vi "main.vi"() -> ()   [LabVIEW 2026]
uses:
  Control/Ctrl_IndicadoresMainPanel.ctl
  Control/Ctr_Enc_Values.ctl
  Control/Ctrl_Motores_Valores.ctl
  Control/Ctrl_Errores.ctl
  Control/Ctrl_DataLoggerQueue.ctl
  Ctrl_Estados.ctl
  Control/Ctrl_EscrituraComandos.ctl
  Control/Ctrl_DLQueue.ctl
  Control/Ctrl_Fgv_DatosMotores.ctl
panel:
  out "Serial errors":u32
  in  "PWM":dbl
  in  "HomeToHome":bool
  in  "Vueltas10":bool
  in  "Serial":refnum<visa-resource-name>
  in  "Refresh Square":bool
  out "status_serial":bool
  out "Start_ind":bool
  in  "Stop Button":bool
  in  "Start Button":bool
  out "Vel_antebrazo":i32 caption="Velocidad"
  out "Vel_hombro":i32 caption="Velocidad"
  out "Vel_mun":i32 caption="Velocidad"
  out "Vel_codo":i32 caption="Velocidad"
  out "Vel_cad":i32 caption="Velocidad"
  out "V_ant":i32 caption="Vueltas"
  out "P_ant":i32 caption="Pasos"
  out "V_hombro":i32 caption="Vueltas"
  out "P_hombro":i32 caption="Pasos"
  out "V_mun":i32 caption="Vueltas"
  out "P_mun":i32 caption="Pasos"
  out "V_cod":i32 caption="Vueltas"
  out "P_cod":i32 caption="Pasos"
  out "V_cad":i32 caption="Vueltas"
  out "P_cad":i32 caption="Pasos"
  out "Enc_Muneca":i32(knob) caption="Enc. Muñeca" scale=0.0..400.0
  out "Error_out":errorcluster
  out "Corriente":dbl
  out "Voltaje":dbl
  out "Enc_Antebrazo":i32(knob) caption="Enc. Antebrazo" scale=0.0..400.0
  out "Enc_Codo":i32(knob) caption="Enc. Codo" scale=0.0..400.0
  out "Enc_Hombro":i32(knob) caption="Enc. Hombro" scale=0.0..400.0
  out "Enc_Cadera":i32(knob) caption="Enc. Cadera" scale=0.0..400.0
  # "Universidad Anáhuac Oaxaca"
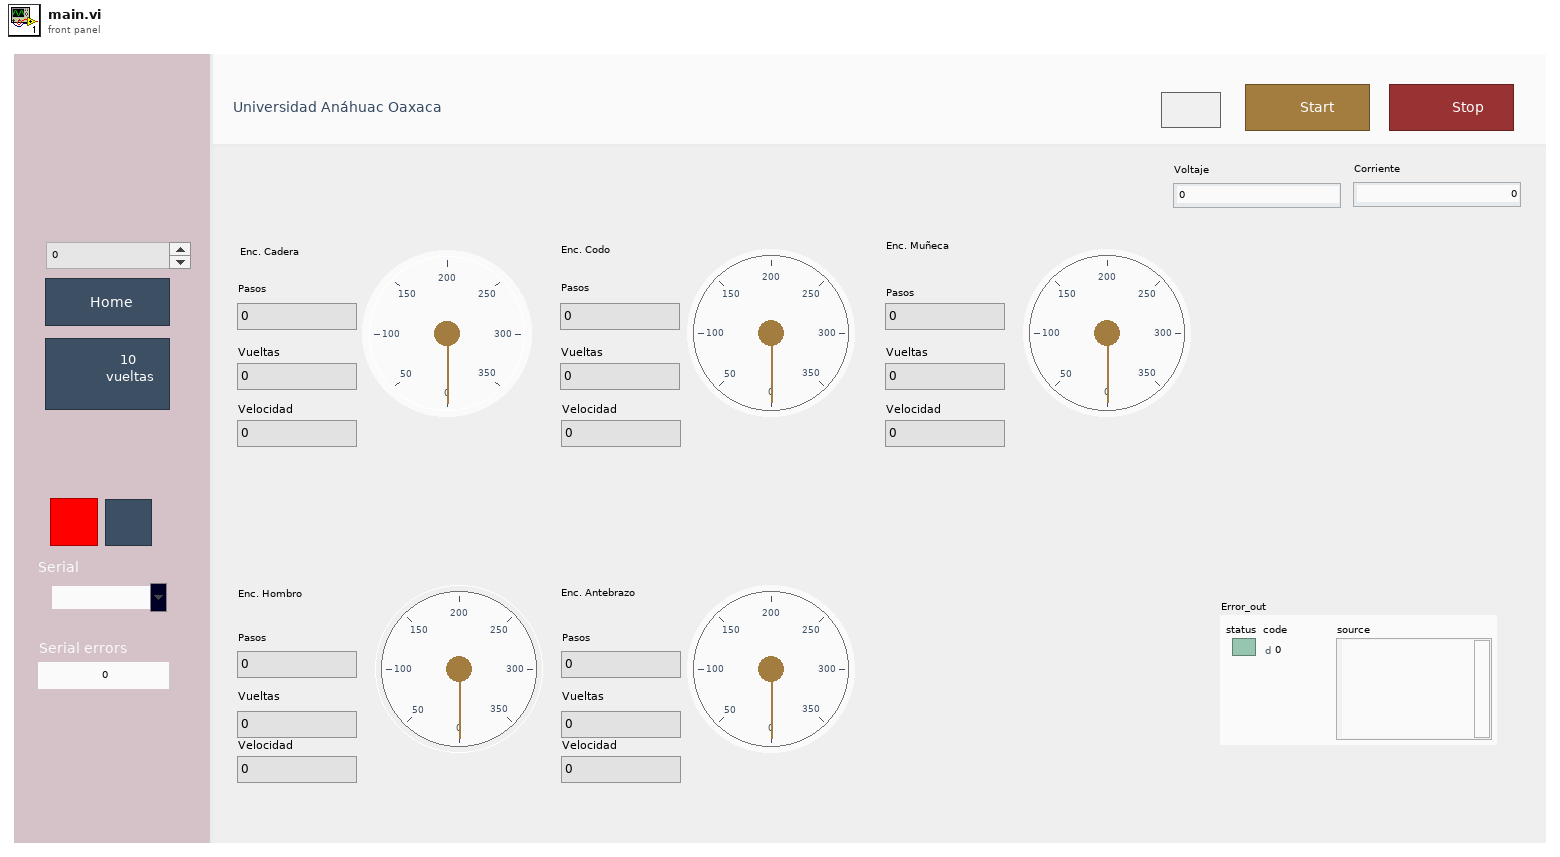
[diagram p1: front panel]
types:
  T1 = enum8{"Enabled", "Disabled", "Disabled and Grayed Out"}
  T2 = typedef "Ctr_Enc_Values.ctl" = cluster{"buffer":string, "Datos6_Motores":cluster{"M_cadera":T3, "M_hombro":T3, "M_codo":T3, "M_antebrazo":T3, "M_muneca":T3, "M_gripper":T3}, "Errores":T4, "new_data?":bool}
  T3 = typedef "Ctrl_Motores_Valores.ctl" = cluster{"Pasos":i32, "Vueltas":i16, "Velocidad":i16, "Reserva1":u8, "Reserva2":u8}
  T4 = typedef "Ctrl_Errores.ctl" = cluster{"Contador_correcto":u32, "Contador_errores":u32, "Edo_conex":u32}
  T5 = typedef "Ctrl_Fgv_DatosMotores.ctl" = enum16{"Stop", "Get", "Set"}
  T6 = typedef "Ctrl_Estados.ctl" = enum16{"LogData", "Idle", "Stop", "IDLE", "Reconnect", "Log_Data_All", "Start", "WRITE_DATA", "SEND_COM"}
  T7 = typedef "Ctrl_DLQueue.ctl" = cluster{"Estado":T6, "IncioPrograma":bool}
  T8 = typedef "Ctrl_DataLoggerQueue.ctl" = cluster{"IncioPrograma":bool, "Estado":T6, "Enc_values":T2, "Com_Escribir":T9}
  T9 = typedef "Ctrl_EscrituraComandos.ctl" = enum16{"MOVE_10", "HOME_TO"}
  T10 = typedef "Ctrl_IndicadoresMainPanel.ctl" = cluster{"status_serial":refnum<vi>, "Vel_cad":refnum<vi>, "Vel_antebrazo":refnum<vi>, "Vel_hombro":refnum<vi>, "Vel_mun":refnum<vi>, "Vel_codo":refnum<vi>, "P_mun":refnum<vi>, "P_ant":refnum<vi>, "P_cod":refnum<vi>, "P_hombro":refnum<vi>, "P_cad":refnum<vi>, "Enc_Antebrazo":refnum<vi>, "Enc_Codo":refnum<vi>, "Enc_Muneca":refnum<vi>, "Enc_Hombro":refnum<vi>, "Enc_Cadera":refnum<vi>, "V_mun":refnum<vi>, "V_ant":refnum<vi>, "V_hombro":refnum<vi>, "V_cod":refnum<vi>, "V_cad":refnum<vi>}
  T11 = enum16{"open", "replace", "create", "open or create", "replace or create", "replace or create with confirmation"}
  T12 = cluster{"M_cadera":T3, "M_hombro":T3, "M_codo":T3, "M_antebrazo":T3, "M_muneca":T3, "M_gripper":T3}
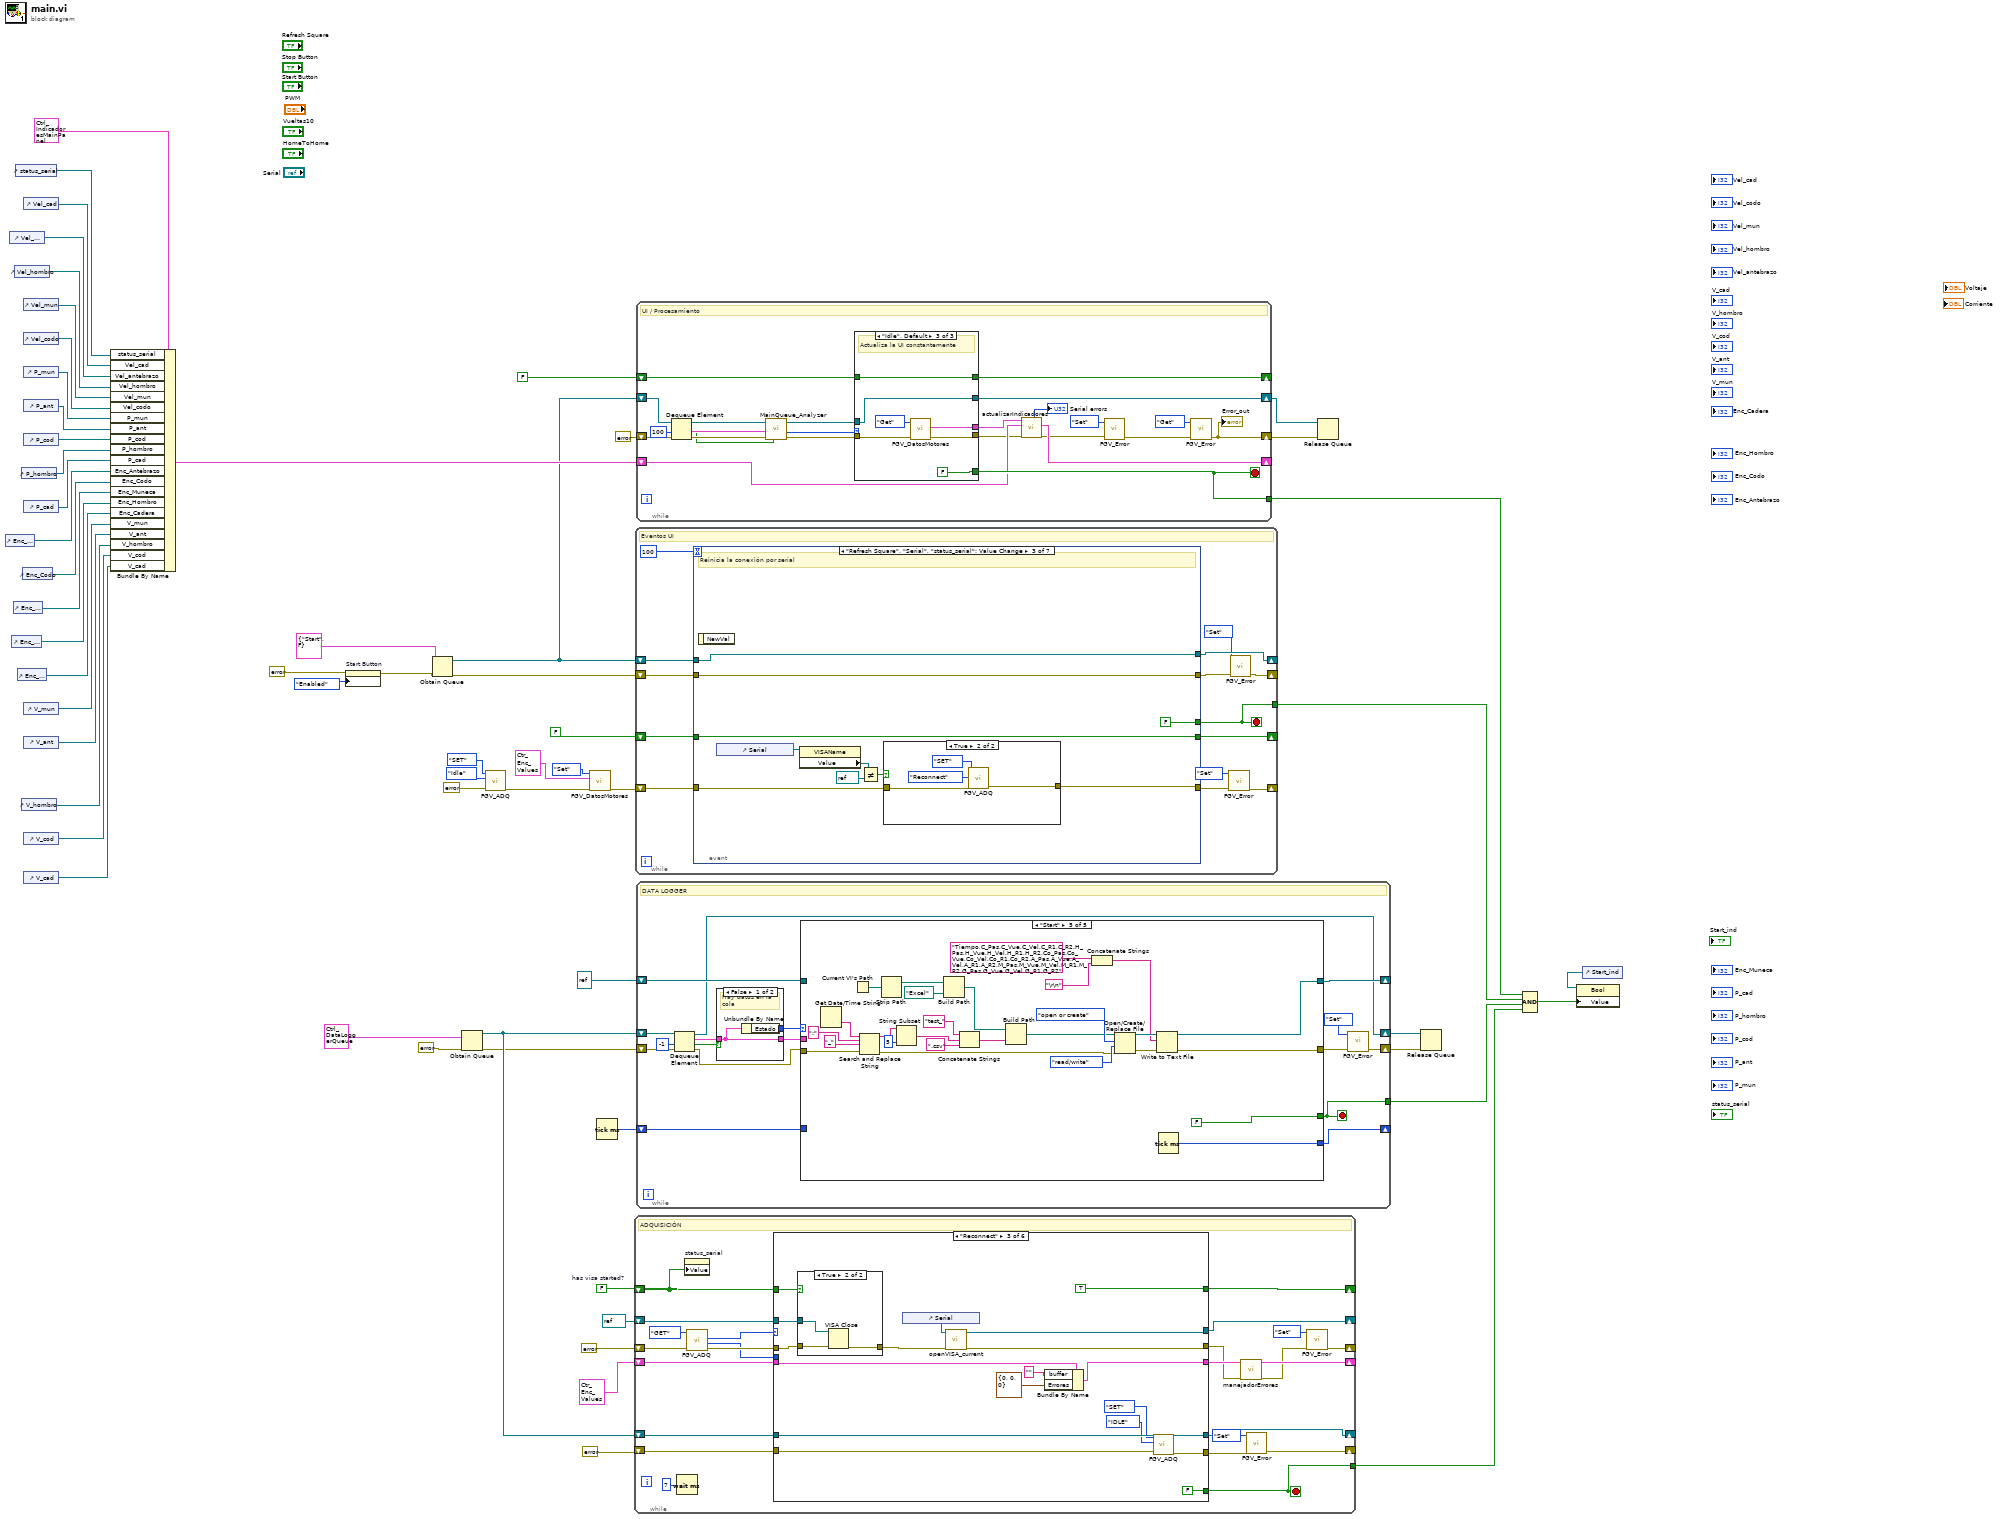
[diagram p0: block diagram]
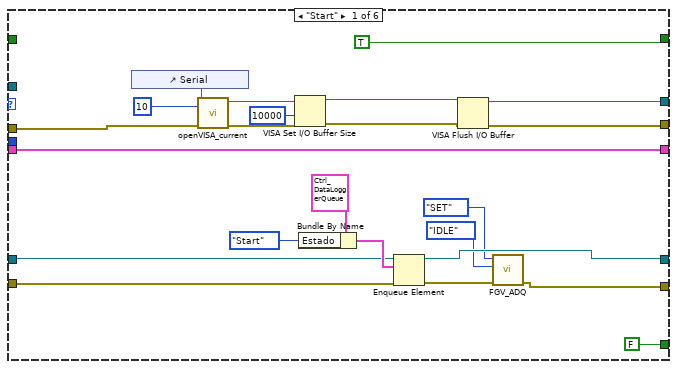
[diagram p2: hidden frame]
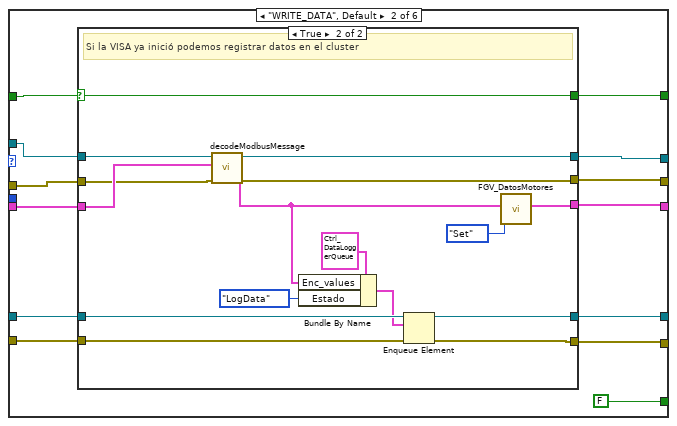
[diagram p3: hidden frame]
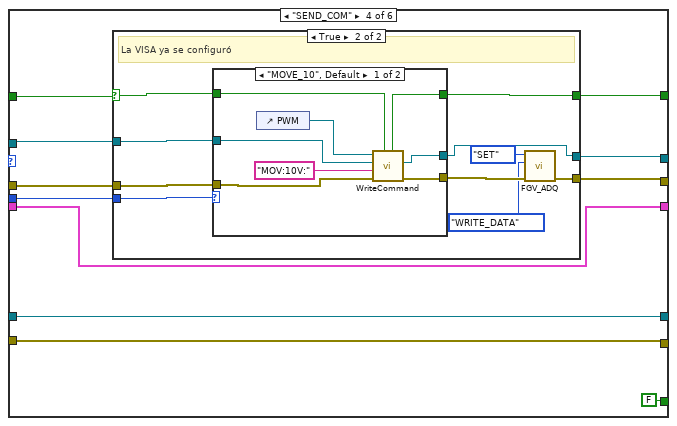
[diagram p6: hidden frame]
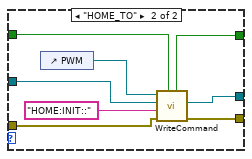
[diagram p8: hidden frame]
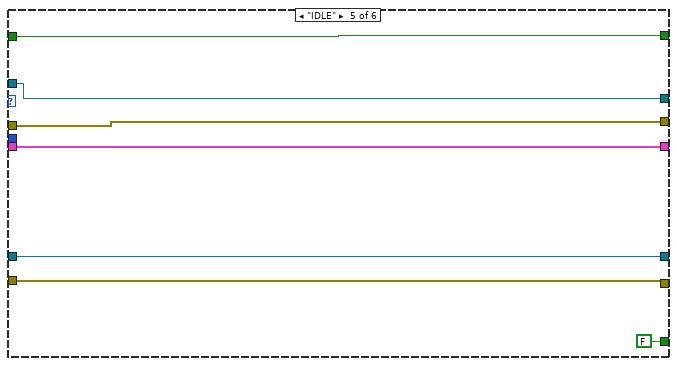
[diagram p9: hidden frame]
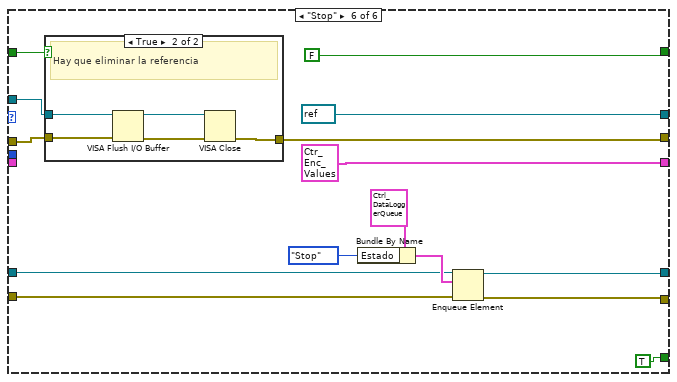
[diagram p10: hidden frame]
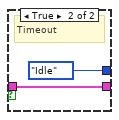
[diagram p12: hidden frame]
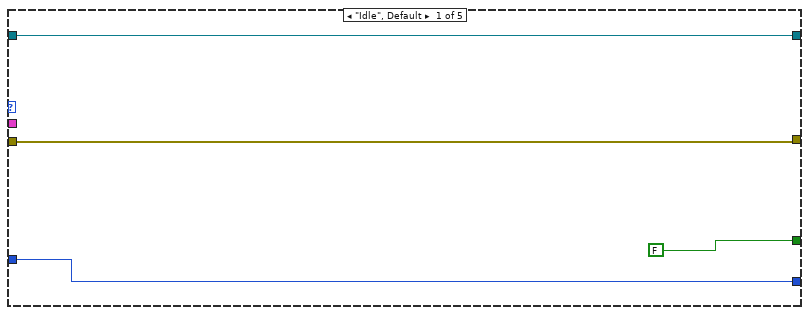
[diagram p13: hidden frame]
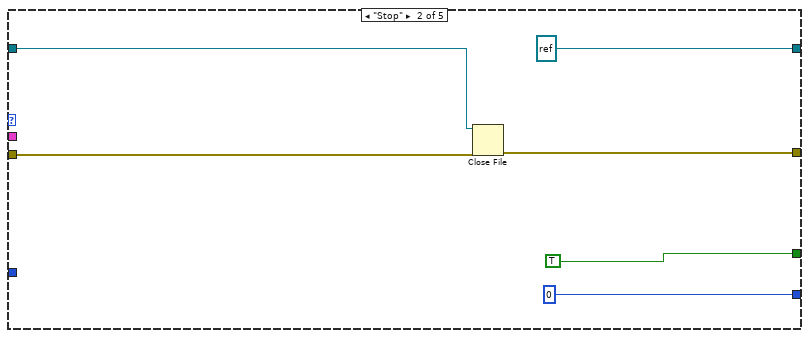
[diagram p14: hidden frame]
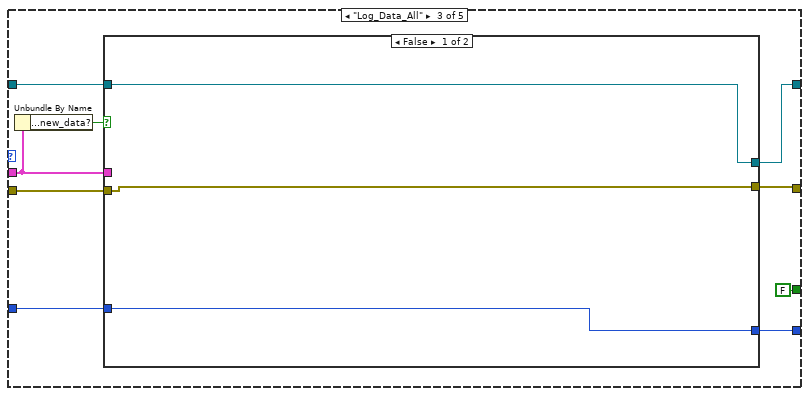
[diagram p15: hidden frame]
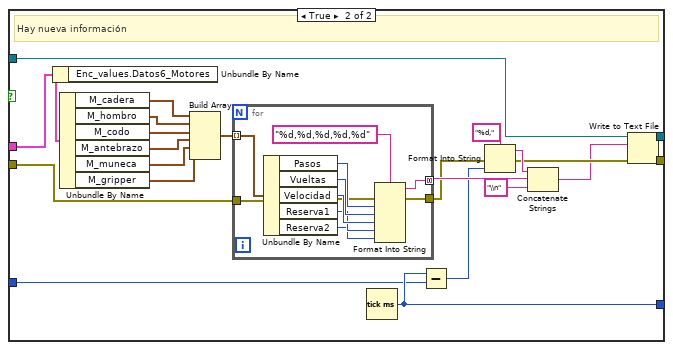
[diagram p16: hidden frame]
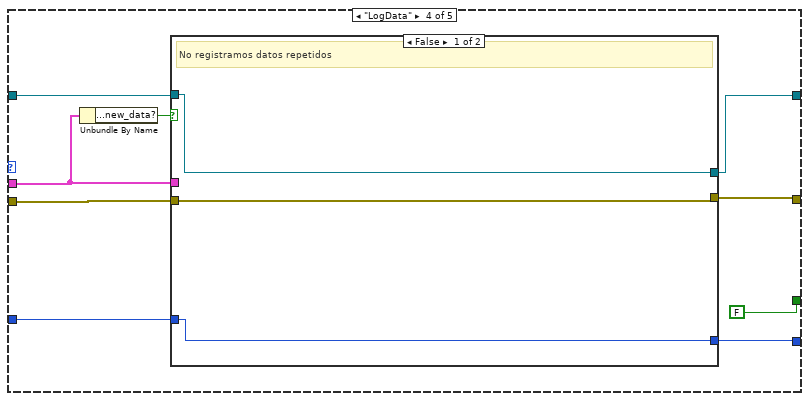
[diagram p17: hidden frame]
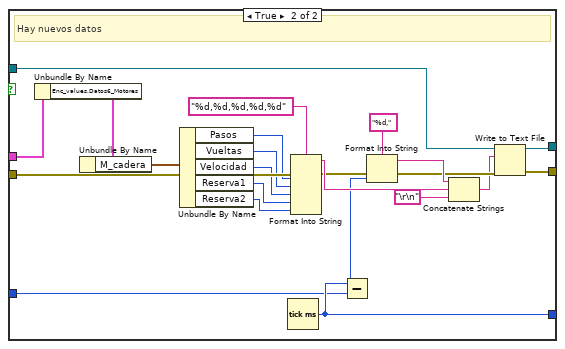
[diagram p18: hidden frame]
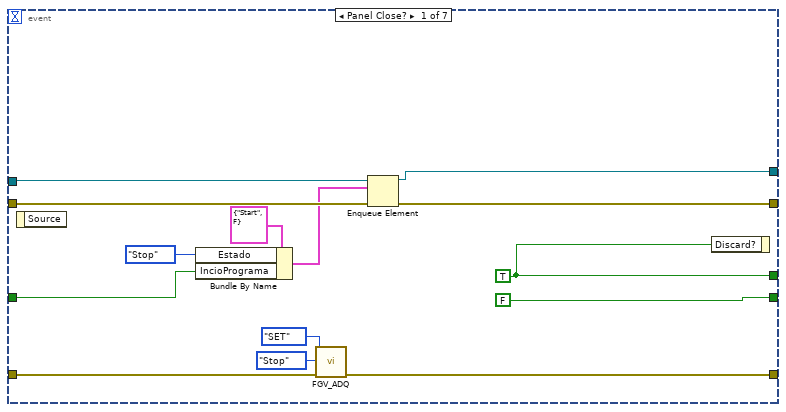
[diagram p19: hidden frame]
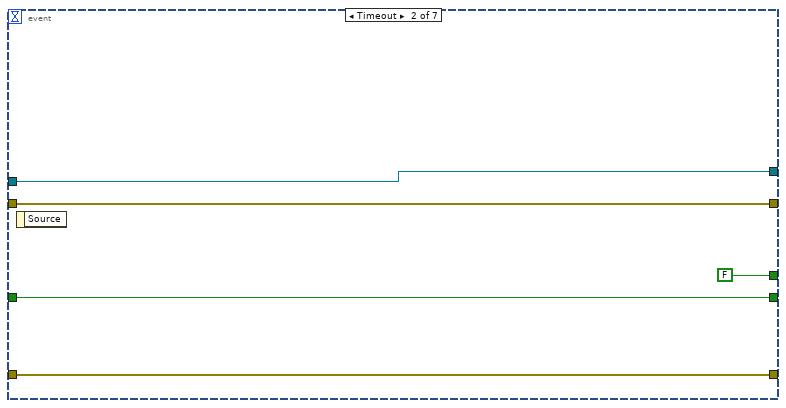
[diagram p20: hidden frame]
diagram:
  w32 = FALSE  # has visa started?
  n1 = control-ref of="Enc_Antebrazo"() -> (w47:refnum<vi>)
  n2 = control-ref of="Vel_antebrazo"() -> (w56:refnum<vi>)
  n3 = control-ref of="Enc_Hombro"() -> (w44:refnum<vi>)
  n4 = control-ref of="Enc_Muneca"() -> (w45:refnum<vi>)
  n5 = control-ref of="Vel_hombro"() -> (w55:refnum<vi>)
  n6 = control-ref of="status_serial"() -> (w59:refnum<vi>)
  n7 = control-ref of="Enc_Cadera"() -> (w43:refnum<vi>)
  n8 = control-ref of="P_hombro"() -> (w49:refnum<vi>)
  n9 = control-ref of="V_hombro"() -> (w40:refnum<vi>)
  n10 = control-ref of="Enc_Codo"() -> (w46:refnum<vi>)
  n11 = control-ref of="Vel_cad"() -> (w57:refnum<vi>)
  n12 = control-ref of="Vel_mun"() -> (w54:refnum<vi>)
  n13 = control-ref of="Vel_codo"() -> (w53:refnum<vi>)
  n14 = control-ref of="P_mun"() -> (w52:refnum<vi>)
  n15 = control-ref of="P_ant"() -> (w51:refnum<vi>)
  n16 = control-ref of="P_cod"() -> (w50:refnum<vi>)
  n17 = control-ref of="P_cad"() -> (w48:refnum<vi>)
  n18 = control-ref of="V_mun"() -> (w42:refnum<vi>)
  n19 = control-ref of="V_ant"() -> (w41:refnum<vi>)
  n20 = control-ref of="V_cod"() -> (w39:refnum<vi>)
  n21 = control-ref of="V_cad"() -> (w38:refnum<vi>)
  n22 = Bundle By Name(cluster=T10 {"status_serial"=refnum, "Vel_cad"=refnum, "Vel_antebrazo"=refnum, "Vel_hombro"=refnum, "Vel_mun"=refnum, "Vel_codo"=refnum, "P_mun"=refnum, "P_ant"=refnum, "P_cod"=refnum, "P_hombro"=refnum, "P_cad"=refnum, "Enc_Antebrazo"=refnum, "Enc_Codo"=refnum, "Enc_Muneca"=refnum, "Enc_Hombro"=refnum, "Enc_Cadera"=refnum, "V_mun"=refnum, "V_ant"=refnum, "V_hombro"=refnum, "V_cod"=refnum, "V_cad"=refnum} ("output cluster"), "status_serial"=w59, "Vel_cad"=w57, "Vel_antebrazo"=w56, "Vel_hombro"=w55, "Vel_mun"=w54, "Vel_codo"=w53, "P_mun"=w52, "P_ant"=w51, "P_cod"=w50, "P_hombro"=w49, "P_cad"=w48, "Enc_Antebrazo"=w47, "Enc_Codo"=w46, "Enc_Muneca"=w45, "Enc_Hombro"=w44, "Enc_Cadera"=w43, "V_mun"=w42, "V_ant"=w41, "V_hombro"=w40, "V_cod"=w39, "V_cad"=w38) -> (w37:T10)
  n23 = property on="Start Button" class="Bool"(error in=errorcluster {"status"=FALSE, "code"=0, "source"=""} ("error in (no error)"), "DisabledEnum"=T1."Enabled" ("Disabled")) -> (error out=w8:errorcluster)  [unwired: 1 in, 1 out]
  n24 = Obtain Queue(element data type=T7 {"Estado"=enum."Start", "IncioPrograma"=FALSE} ("estado_queue"), error in (no error)=w8) -> (queue out=w22:refnum<queue>, error out=w21:errorcluster)  [unwired: 3 in, 1 out]
  n25 = Obtain Queue(element data type=T8 {"IncioPrograma"=FALSE, "Estado"=enum."Start", "Enc_values"={"buffer"="", "Datos6_Motores"={"M_cadera"={"Pasos"=0, "Vueltas"=0, "Velocidad"=0, "Reserva1"=0, "Reserva2"=0}, "M_hombro"={"Pasos"=0, "Vueltas"=0, "Velocidad"=0, "Reserva1"=0, "Reserva2"=0}, "M_codo"={"Pasos"=0, "Vueltas"=0, "Velocidad"=0, "Reserva1"=0, "Reserva2"=0}, "M_antebrazo"={"Pasos"=0, "Vueltas"=0, "Velocidad"=0, "Reserva1"=0, "Reserva2"=0}, "M_muneca"={"Pasos"=0, "Vueltas"=0, "Velocidad"=0, "Reserva1"=0, "Reserva2"=0}, "M_gripper"={"Pasos"=0, "Vueltas"=0, "Velocidad"=0, "Reserva1"=0, "Reserva2"=0}}, "Errores"={"Contador_correcto"=0, "Contador_errores"=0, "Edo_conex"=0}, "new_data?"=FALSE}, "Com_Escribir"=enum."MOVE_10"} ("datalogger_cluster"), error in (no error)=errorcluster {"status"=FALSE, "code"=0, "source"=""}) -> (queue out=w10:refnum<queue>, error out=w9:errorcluster)  [unwired: 3 in, 1 out]
  n26 = call "FGV_ADQ.vi"("error in (no error)"=errorcluster {"status"=FALSE, "code"=0, "source"=""}, "SM_IN"=Ctrl_Estados."Idle", "SET/GET"=enum16{"SET", "GET"}."SET") -> ("error out"=w11:errorcluster)  [unwired: 6 in, 2 out]
  n27 = call "FGV_DatosMotores.vi"("error in (no error)"=w11, "Val_motor_in"=T2 {"buffer"="", "Datos6_Motores"={"M_cadera"={"Pasos"=0, "Vueltas"=0, "Velocidad"=0, "Reserva1"=0, "Reserva2"=0}, "M_hombro"={"Pasos"=0, "Vueltas"=0, "Velocidad"=0, "Reserva1"=0, "Reserva2"=0}, "M_codo"={"Pasos"=0, "Vueltas"=0, "Velocidad"=0, "Reserva1"=0, "Reserva2"=0}, "M_antebrazo"={"Pasos"=0, "Vueltas"=0, "Velocidad"=0, "Reserva1"=0, "Reserva2"=0}, "M_muneca"={"Pasos"=0, "Vueltas"=0, "Velocidad"=0, "Reserva1"=0, "Reserva2"=0}, "M_gripper"={"Pasos"=0, "Vueltas"=0, "Velocidad"=0, "Reserva1"=0, "Reserva2"=0}}, "Errores"={"Contador_correcto"=0, "Contador_errores"=0, "Edo_conex"=0}, "new_data?"=FALSE}, "Estado"=Ctrl_Fgv_DatosMotores."Set") -> ("error out"=w14:errorcluster)  [unwired: 7 in, 1 out]
  n28 = Tick Count (ms)() -> (millisecond timer value=w36:u32)
  n29 = while {
    shift-right: [w75] -> _
    shift-left: T2 {"buffer"="", "Datos6_Motores"={"M_cadera"={"Pasos"=0, "Vueltas"=0, "Velocidad"=0, "Reserva1"=0, "Reserva2"=0}, "M_hombro"={"Pasos"=0, "Vueltas"=0, "Velocidad"=0, "Reserva1"=0, "Reserva2"=0}, "M_codo"={"Pasos"=0, "Vueltas"=0, "Velocidad"=0, "Reserva1"=0, "Reserva2"=0}, "M_antebrazo"={"Pasos"=0, "Vueltas"=0, "Velocidad"=0, "Reserva1"=0, "Reserva2"=0}, "M_muneca"={"Pasos"=0, "Vueltas"=0, "Velocidad"=0, "Reserva1"=0, "Reserva2"=0}, "M_gripper"={"Pasos"=0, "Vueltas"=0, "Velocidad"=0, "Reserva1"=0, "Reserva2"=0}}, "Errores"={"Contador_correcto"=0, "Contador_errores"=0, "Edo_conex"=0}, "new_data?"=FALSE} ("Enc_values") -> [w84]
    shift-right: [w83] -> _
    shift-left: refnum<visa-resource-name> refnum ("VISA resource name out") -> [w81]
    shift-right: [w71] -> _
    shift-left: errorcluster {"status"=FALSE, "code"=0, "source"=""} ("error in (no error)") -> [w67]
    shift-right: [w82] -> _
    shift-left: w32 -> [w62]
    shift-right: [w64] -> _
    shift-left: errorcluster {"status"=FALSE, "code"=0, "source"=""} ("error in (no error)") -> [w80]
    shift-right: [w78] -> _
    shift-left: w10 -> [w79]
    tunnel: [w77] -> w24
    stop <- w77 stop-if-true
    # "ADQUISICIÓN"
    n30 = Wait (ms)(milliseconds to wait=u32 7) -> ()  [unwired: 1 out]
    n31 = property on="status_serial" class="Bool"("Value"=w62) -> ()  [unwired: 2 in, 2 out]
    n32 = call "FGV_ADQ.vi"("error in (no error)"=w67, "SET/GET"=enum16{"SET", "GET"}."GET") -> ("error out"=w68:errorcluster, "Com_Escribir_OUT"=w66:T9, "SM_OUT"=w69:T6)  [unwired: 7 in]
    n33 = case shown="\"Reconnect\"" w69 {
      tunnel: w84 -> [w106 w120 w154 w172 w208 _]
      tunnel: w81 -> [_ w119 w157 w175 w210 w225]
      tunnel: w62 -> [_ w117 w152 w170 w211 w226]
      tunnel: [w88 w110 w155 w174 w209 w221] -> w74
      tunnel: [w89 w118 w150 w171 w210 refnum<visa-resource-name> refnum ("VISA resource name out")] -> w83
      tunnel: [TRUE w113 TRUE ("start_out") w173 w211 FALSE] -> w82
      tunnel: [w106 w111 w153 w172 w208 T2 {"buffer"="", "Datos6_Motores"={"M_cadera"={"Pasos"=0, "Vueltas"=0, "Velocidad"=0, "Reserva1"=0, "Reserva2"=0}, "M_hombro"={"Pasos"=0, "Vueltas"=0, "Velocidad"=0, "Reserva1"=0, "Reserva2"=0}, "M_codo"={"Pasos"=0, "Vueltas"=0, "Velocidad"=0, "Reserva1"=0, "Reserva2"=0}, "M_antebrazo"={"Pasos"=0, "Vueltas"=0, "Velocidad"=0, "Reserva1"=0, "Reserva2"=0}, "M_muneca"={"Pasos"=0, "Vueltas"=0, "Velocidad"=0, "Reserva1"=0, "Reserva2"=0}, "M_gripper"={"Pasos"=0, "Vueltas"=0, "Velocidad"=0, "Reserva1"=0, "Reserva2"=0}}, "Errores"={"Contador_correcto"=0, "Contador_errores"=0, "Edo_conex"=0}, "new_data?"=FALSE} ("Enc_values")] -> w76
      tunnel: w80 -> [w101 w116 w143 w165 w205 w216]
      tunnel: w79 -> [w102 w115 w149 w169 w207 w217]
      tunnel: [w100 w114 w149 w169 w207 w215] -> w78
      tunnel: [FALSE FALSE FALSE FALSE FALSE TRUE] -> w77
      tunnel: w68 -> [w98 w109 w147 w167 w209 w213]
      tunnel: w66 -> [_ _ _ w166 _ _]
      tunnel: [w85 w108 w144 w165 w205 w212] -> w61
      frame "Start" {
        n34 = control-ref of="Serial"() -> (w107:refnum<vi>)
        n35 = call "openVISA_current.vi"("error in (no error)"=w98, "Timeout"=u32 10, "VisaRef"=w107) -> ("error out"=w92:errorcluster, "VISA Refnum out"=w93:refnum<visa-resource-name>)  [unwired: 7 in]
        n36 = VISA Set I/O Buffer Size(VISA resource name=w93, size (4096)=u32 10000, error in (no error)=w92) -> (VISA resource name out=w91:refnum<visa-resource-name>, error out=w90:errorcluster)  [unwired: 1 in]
        n37 = Bundle By Name(cluster=T8 {"IncioPrograma"=FALSE, "Estado"=enum."Start", "Enc_values"={"buffer"="", "Datos6_Motores"={"M_cadera"={"Pasos"=0, "Vueltas"=0, "Velocidad"=0, "Reserva1"=0, "Reserva2"=0}, "M_hombro"={"Pasos"=0, "Vueltas"=0, "Velocidad"=0, "Reserva1"=0, "Reserva2"=0}, "M_codo"={"Pasos"=0, "Vueltas"=0, "Velocidad"=0, "Reserva1"=0, "Reserva2"=0}, "M_antebrazo"={"Pasos"=0, "Vueltas"=0, "Velocidad"=0, "Reserva1"=0, "Reserva2"=0}, "M_muneca"={"Pasos"=0, "Vueltas"=0, "Velocidad"=0, "Reserva1"=0, "Reserva2"=0}, "M_gripper"={"Pasos"=0, "Vueltas"=0, "Velocidad"=0, "Reserva1"=0, "Reserva2"=0}}, "Errores"={"Contador_correcto"=0, "Contador_errores"=0, "Edo_conex"=0}, "new_data?"=FALSE}, "Com_Escribir"=enum."MOVE_10"} ("datalogger_cluster"), "Estado"=Ctrl_Estados."Start") -> (w104:T8)
        n38 = Enqueue Element(queue=w102, element=w104, error in (no error)=w101) -> (queue out=w100:refnum<queue>, error out=w96:errorcluster)  [unwired: 1 in, 1 out]
        n39 = VISA Flush I/O Buffer(VISA resource name=w91, error in (no error)=w90) -> (VISA resource name out=w89:refnum<visa-resource-name>, error out=w88:errorcluster)  [unwired: 1 in]
        n40 = call "FGV_ADQ.vi"("error in (no error)"=w96, "SM_IN"=Ctrl_Estados."IDLE", "SET/GET"=enum16{"SET", "GET"}."SET") -> ("error out"=w85:errorcluster)  [unwired: 6 in, 2 out]
      }
      frame "WRITE_DATA", Default {
        n41 = case shown="True" w117 {
          selector: w117 -> [w122 w130]
          tunnel: w120 -> [w125 w140]
          tunnel: w119 -> [w126 w139]
          tunnel: [w125 w129] -> w111
          tunnel: [w121 w128] -> w110
          tunnel: [w126 w138] -> w118
          tunnel: w116 -> [w123 w137]
          tunnel: w115 -> [w124 w136]
          tunnel: [w123 w133] -> w108
          tunnel: [w124 w132] -> w114
          tunnel: [w122 w130] -> w113
          tunnel: w109 -> [w121 w127]
          frame False {
            # "Si la VISA no ha iniciado no es posible leer del serial"
          }
          frame True {
            # "Si la VISA ya inició podemos registrar datos en el cluster"
            n42 = call "decodeModbusMessage.vi"("error in (no error)"=w127, "Enc_values_in"=w140, "VISA resource name"=w139) -> ("error out"=w128:errorcluster, "Enc_values_out 2"=w134:T2, "VISA Refnum out"=w138:refnum<visa-resource-name>)  [unwired: 6 in]
            n43 = Bundle By Name(cluster=T8 {"IncioPrograma"=FALSE, "Estado"=enum."Start", "Enc_values"={"buffer"="", "Datos6_Motores"={"M_cadera"={"Pasos"=0, "Vueltas"=0, "Velocidad"=0, "Reserva1"=0, "Reserva2"=0}, "M_hombro"={"Pasos"=0, "Vueltas"=0, "Velocidad"=0, "Reserva1"=0, "Reserva2"=0}, "M_codo"={"Pasos"=0, "Vueltas"=0, "Velocidad"=0, "Reserva1"=0, "Reserva2"=0}, "M_antebrazo"={"Pasos"=0, "Vueltas"=0, "Velocidad"=0, "Reserva1"=0, "Reserva2"=0}, "M_muneca"={"Pasos"=0, "Vueltas"=0, "Velocidad"=0, "Reserva1"=0, "Reserva2"=0}, "M_gripper"={"Pasos"=0, "Vueltas"=0, "Velocidad"=0, "Reserva1"=0, "Reserva2"=0}}, "Errores"={"Contador_correcto"=0, "Contador_errores"=0, "Edo_conex"=0}, "new_data?"=FALSE}, "Com_Escribir"=enum."MOVE_10"} ("datalogger_cluster"), "Enc_values"=w134, "Estado"=Ctrl_Estados."LogData") -> (w135:T8)
            n44 = Enqueue Element(queue=w136, element=w135, error in (no error)=w137) -> (queue out=w132:refnum<queue>, error out=w133:errorcluster)  [unwired: 1 in, 1 out]
            n45 = call "FGV_DatosMotores.vi"("Val_motor_in"=w134, "Estado"=Ctrl_Fgv_DatosMotores."Set") -> ("Val_motor_out"=w129:T2)  [unwired: 8 in, 1 out]
          }
        }
      }
      frame "Reconnect" {
        n46 = case shown="True" w152 {
          tunnel: [w161 w164] -> w158
          tunnel: w157 -> [_ w163]
          tunnel: w147 -> [w161 w162]
          frame False {
          }
          frame True {
            n47 = VISA Close(VISA resource name=w163, error in (no error)=w162) -> (error out=w164:errorcluster)
          }
        }
        n48 = control-ref of="Serial"() -> (w156:refnum<vi>)
        n49 = call "openVISA_current.vi"("error in (no error)"=w158, "VisaRef"=w156) -> ("error out"=w155:errorcluster, "VISA Refnum out"=w150:refnum<visa-resource-name>)  [unwired: 8 in]
        n50 = Bundle By Name(cluster=w154, "buffer"="", "Errores"=T4 {"Contador_correcto"=0, "Contador_errores"=0, "Edo_conex"=0}) -> (w153:T2)
        n51 = call "FGV_ADQ.vi"("error in (no error)"=w143, "SM_IN"=Ctrl_Estados."IDLE", "SET/GET"=enum16{"SET", "GET"}."SET") -> ("error out"=w144:errorcluster)  [unwired: 6 in, 2 out]
      }
      frame "SEND_COM" {
        n52 = case shown="True" w170 {
          selector: w170 -> [w177 w185]
          tunnel: w175 -> [w178 w188]
          tunnel: [w176 w182] -> w174
          tunnel: [w177 w187] -> w173
          tunnel: [w178 w186] -> w171
          tunnel: w167 -> [w176 w184]
          tunnel: w166 -> [_ w183]
          frame False {
            # "La VISA no se ha configurado"
          }
          frame True {
            # "La VISA ya se configuró"
            n53 = case shown="\"MOVE_10\", Default" w183 {
              tunnel: w188 -> [w194 w203]
              tunnel: [w195 w201] -> w181
              tunnel: w185 -> [w192 w200]
              tunnel: [w191 w199] -> w187
              tunnel: [w193 w198] -> w186
              tunnel: w184 -> [w189 w197]
              frame "MOVE_10", Default {
                n54 = control-ref of="PWM"() -> (w190:refnum<vi>)
                n55 = call "WriteCommand.vi"("start_in"=w192, "errorI_n_interface"=w189, "write buffer"="MOV:10V:", "VISA resource name"=w194, "PWM 2"=w190) -> ("error_out_interface"=w195:errorcluster, "VISA resource name 2"=w193:refnum<visa-resource-name>, "start_out"=w191:bool)  [unwired: 4 in]
              }
              frame "HOME_TO" {
                n56 = control-ref of="PWM"() -> (w202:refnum<vi>)
                n57 = call "WriteCommand.vi"("start_in"=w200, "errorI_n_interface"=w197, "write buffer"="HOME:INIT::", "VISA resource name"=w203, "PWM 2"=w202) -> ("error_out_interface"=w201:errorcluster, "VISA resource name 2"=w198:refnum<visa-resource-name>, "start_out"=w199:bool)  [unwired: 4 in]
              }
            }
            n58 = call "FGV_ADQ.vi"("error in (no error)"=w181, "SM_IN"=Ctrl_Estados."WRITE_DATA", "SET/GET"=enum16{"SET", "GET"}."SET") -> ("error out"=w182:errorcluster)  [unwired: 6 in, 2 out]
          }
        }
      }
      frame "IDLE" {
      }
      frame "Stop" {
        n59 = case shown="True" w226 {
          tunnel: w225 -> [_ w229]
          tunnel: [w227 w232] -> w221
          tunnel: w213 -> [w227 w230]
          frame False {
          }
          frame True {
            # "Hay que eliminar la referencia"
            n60 = VISA Flush I/O Buffer(VISA resource name=w229, error in (no error)=w230) -> (VISA resource name out=w228:refnum<visa-resource-name>, error out=w231:errorcluster)  [unwired: 1 in]
            n61 = VISA Close(VISA resource name=w228, error in (no error)=w231) -> (error out=w232:errorcluster)
          }
        }
        n62 = Bundle By Name(cluster=T8 {"IncioPrograma"=FALSE, "Estado"=enum."Start", "Enc_values"={"buffer"="", "Datos6_Motores"={"M_cadera"={"Pasos"=0, "Vueltas"=0, "Velocidad"=0, "Reserva1"=0, "Reserva2"=0}, "M_hombro"={"Pasos"=0, "Vueltas"=0, "Velocidad"=0, "Reserva1"=0, "Reserva2"=0}, "M_codo"={"Pasos"=0, "Vueltas"=0, "Velocidad"=0, "Reserva1"=0, "Reserva2"=0}, "M_antebrazo"={"Pasos"=0, "Vueltas"=0, "Velocidad"=0, "Reserva1"=0, "Reserva2"=0}, "M_muneca"={"Pasos"=0, "Vueltas"=0, "Velocidad"=0, "Reserva1"=0, "Reserva2"=0}, "M_gripper"={"Pasos"=0, "Vueltas"=0, "Velocidad"=0, "Reserva1"=0, "Reserva2"=0}}, "Errores"={"Contador_correcto"=0, "Contador_errores"=0, "Edo_conex"=0}, "new_data?"=FALSE}, "Com_Escribir"=enum."MOVE_10"} ("datalogger_cluster"), "Estado"=Ctrl_Estados."Stop") -> (w219:T8)
        n63 = Enqueue Element(queue=w217, element=w219, error in (no error)=w216) -> (queue out=w215:refnum<queue>, error out=w212:errorcluster)  [unwired: 1 in, 1 out]
      }
    }
    n64 = call "manejadorErrores.vi"("error in (no error)"=w74, "Enc_values"=w76) -> ("error out"=w72:errorcluster, "Enc_values 2"=w75:T2)  [unwired: 8 in]
    n65 = call "FGV_Error.vi"("error_in_loop"=w61, "Estado"=enum16{"Set", "Get"}."Set") -> ("error out"=w64:errorcluster)  [unwired: 9 in]
    n66 = call "FGV_Error.vi"("error_in_loop"=w72, "Estado"=enum16{"Set", "Get"}."Set") -> ("error out"=w71:errorcluster)  [unwired: 9 in]
  }
  n67 = while {
    shift-right: [w240] -> _
    shift-left: FALSE -> [w243]
    shift-right: [w241] -> _
    shift-left: w22 -> [w244]
    shift-right: [w237] -> _
    shift-left: w21 -> [w245]
    shift-right: [w233] -> _
    shift-left: w14 -> [w242]
    tunnel: [w239] -> w27
    stop <- w239 stop-if-true
    # "Eventos UI"
    n68 = event shown="[2] \"Refresh Square\", \"Serial\", \"status_serial\": Value Change" {
      selector: _ -> [_ _ _ _ _ _ _]
      dyn-events: _ -> [_ _ _ _ _ _ _]
      timeout: 100 -> [_ _ _ _ _ _ _]
      tunnel: [w257 FALSE FALSE FALSE FALSE FALSE TRUE] -> w239
      tunnel: w245 -> [w259 w265 w274 w286 w295 w309 w339]
      tunnel: [w260 w265 w274 w286 w295 w313 w340] -> w236
      tunnel: w244 -> [w258 w264 w270 w287 w296 w311 w338]
      tunnel: [w247 w264 w270 w287 w296 w312 w327] -> w241
      tunnel: w243 -> [w253 w262 w275 w289 w298 _ w334]
      tunnel: [FALSE w262 w275 w289 w298 w300 FALSE] -> w240
      tunnel: w242 -> [w251 w261 w272 w282 w290 w303 w328]
      tunnel: [w248 w261 w271 w281 w291 w302 w329] -> w234
      event Panel Close? {
        w257 = TRUE
        n69 = event-data() -> ()  [unwired: 1 in, 1 out]
        n70 = Bundle By Name(cluster=T7 {"Estado"=enum."Start", "IncioPrograma"=FALSE} ("estado_queue"), "Estado"=Ctrl_Estados."Stop", "IncioPrograma"=w253) -> (w254:T7)
        n71 = call "FGV_ADQ.vi"("error in (no error)"=w251, "SM_IN"=Ctrl_Estados."Stop", "SET/GET"=enum16{"SET", "GET"}."SET") -> ("error out"=w248:errorcluster)  [unwired: 6 in, 2 out]
        n72 = Enqueue Element(queue=w258, element=w254, error in (no error)=w259) -> (queue out=w247:refnum<queue>, error out=w260:errorcluster)  [unwired: 1 in, 1 out]
        n73 = event-data("Discard?"=w257) -> ()  [unwired: 1 in, 1 out]
      }
      event Timeout {
        n74 = event-data() -> ()  [unwired: 1 in, 1 out]
      }
      event "Refresh Square", "Serial", "status_serial": Value Change {
        # "Reinicia la conexión por serial"
        n75 = event-data() -> ()  [unwired: 1 in, 1 out]
        n76 = control-ref of="Serial"() -> (w269:refnum<vi>)
        n77 = property class="VISAName"(reference=w269) -> ("Value"=w267:refnum<visa-resource-name>)  [unwired: 1 in, 2 out]
        n78 = Not Equal?(x=w267, y=refnum<visa-resource-name> refnum) -> (x != y?=w268:bool)
        n79 = case shown="True" w268 {
          tunnel: w272 -> [w276 w278]
          tunnel: [w276 w277] -> w271
          frame False {
          }
          frame True {
            n80 = call "FGV_ADQ.vi"("error in (no error)"=w278, "SM_IN"=Ctrl_Estados."Reconnect", "SET/GET"=enum16{"SET", "GET"}."SET") -> ("error out"=w277:errorcluster)  [unwired: 6 in, 2 out]
          }
        }
      }
      event "HomeToHome": Value Change {
        n81 = event-data() -> ()  [unwired: 1 in, 1 out]
        n82 = call "FGV_ADQ.vi"("error in (no error)"=w282, "Com_Escribir_IN"=Ctrl_EscrituraComandos."HOME_TO", "SM_IN"=Ctrl_Estados."SEND_COM", "SET/GET"=enum16{"SET", "GET"}."SET") -> ("error out"=w281:errorcluster)  [unwired: 5 in, 2 out]
      }
      event "Vueltas10": Value Change {
        n83 = event-data() -> ()  [unwired: 1 in, 1 out]
        n84 = call "FGV_ADQ.vi"("error in (no error)"=w290, "Com_Escribir_IN"=Ctrl_EscrituraComandos."MOVE_10", "SM_IN"=Ctrl_Estados."SEND_COM", "SET/GET"=enum16{"SET", "GET"}."SET") -> ("error out"=w291:errorcluster)  [unwired: 5 in, 2 out]
      }
      event "Start Button": Value Change {
        n85 = event-data() -> ()  [unwired: 1 in, 1 out]
        n86 = control-ref of="Serial"() -> (w304:refnum<vi>)
        n87 = property class="VISAName"(reference=w304, error in=w309) -> (error out=w299:errorcluster, "Value"=w308:refnum<visa-resource-name>)  [unwired: 1 out]
        n88 = Not Equal?(x=w308, y=refnum<visa-resource-name> refnum) -> (x != y?=w305:bool)
        n89 = case shown="True" w305 {
          selector: w305 -> [w316 w325]
          tunnel: [w316 w325] -> w300
          tunnel: [Ctrl_Estados."Idle" Ctrl_Estados."Start"] -> w306
          tunnel: w303 -> [w317 w322]
          tunnel: [w317 w323] -> w302
          frame False {
          }
          frame True {
            n90 = property on="Start Button" class="Bool"(error in=w322, "DisabledEnum"=T1."Disabled" ("Disabled")) -> (error out=w321:errorcluster)  [unwired: 1 in, 1 out]
            n91 = call "FGV_ADQ.vi"("error in (no error)"=w321, "SM_IN"=Ctrl_Estados."Start", "SET/GET"=enum16{"SET", "GET"}."SET") -> ("error out"=w323:errorcluster)  [unwired: 6 in, 2 out]
          }
        }
        n92 = Bundle By Name(cluster=T7 {"Estado"=enum."Start", "IncioPrograma"=FALSE} ("estado_queue"), "Estado"=w306) -> (w314:T7)
        n93 = control-ref of="Start_ind"() -> (w301:refnum<vi>)
        n94 = property class="Bool"(reference=w301, "Value"=w300) -> ()  [unwired: 1 in, 2 out]
        n95 = Enqueue Element(queue=w311, element=w314, error in (no error)=w299) -> (queue out=w312:refnum<queue>, error out=w313:errorcluster)  [unwired: 1 in, 1 out]
      }
      event "Stop Button": Value Change {
        n96 = event-data() -> ()  [unwired: 1 in, 1 out]
        n97 = Bundle By Name(cluster=T7 {"Estado"=enum."Start", "IncioPrograma"=FALSE} ("estado_queue"), "Estado"=Ctrl_Estados."Stop", "IncioPrograma"=w334) -> (w335:T7)
        n98 = Enqueue Element(queue=w338, element=w335, error in (no error)=w339) -> (queue out=w327:refnum<queue>, error out=w340:errorcluster)  [unwired: 1 in, 1 out]
        n99 = call "FGV_ADQ.vi"("error in (no error)"=w328, "SM_IN"=Ctrl_Estados."Stop", "SET/GET"=enum16{"SET", "GET"}."SET") -> ("error out"=w329:errorcluster)  [unwired: 6 in, 2 out]
      }
    }
    n100 = call "FGV_Error.vi"("error_in_loop"=w234, "Estado"=enum16{"Set", "Get"}."Set") -> ("error out"=w233:errorcluster)  [unwired: 9 in]
    n101 = call "FGV_Error.vi"("error_in_loop"=w236, "Estado"=enum16{"Set", "Get"}."Set") -> ("error out"=w237:errorcluster)  [unwired: 9 in]
  }
  n102 = while {
    shift-right: [w342] -> w17
    shift-left: errorcluster {"status"=FALSE, "code"=0, "source"=""} ("error out") -> [w364]
    shift-right: [w350] -> w18
    shift-left: w22 -> [w363]
    shift-right: [w353] -> _
    shift-left: w37 -> [w352]
    tunnel: [w356] -> w25
    shift-right: [w347] -> _
    shift-left: FALSE -> [w349]
    stop <- w356 stop-if-true
    # "UI / Procesamiento"
    n103 = Dequeue Element(queue=w363, timeout in ms (-1)=100, error in (no error)=w364) -> (queue out=w361:refnum<queue>, element=w358:T7, timed out?=w355:bool, error out=w360:errorcluster)
    n104 = call "MainQueue_Analyzer.vi"("timed out?"=w355, "error in (no error)"=w360, "estado_queue"=w358, "Queue in"=w361) -> ("error out"=w359:errorcluster, "Estado"=w357:T6, "Queue out"=w351:refnum<queue>)  [unwired: 4 in, 1 out]
    n105 = case shown="\"Idle\", Default" w357 {
      tunnel: w359 -> [w366 w370 w375]
      tunnel: [FALSE TRUE FALSE] -> w356
      tunnel: [T2 {"buffer"="", "Datos6_Motores"={"M_cadera"={"Pasos"=0, "Vueltas"=0, "Velocidad"=0, "Reserva1"=0, "Reserva2"=0}, "M_hombro"={"Pasos"=0, "Vueltas"=0, "Velocidad"=0, "Reserva1"=0, "Reserva2"=0}, "M_codo"={"Pasos"=0, "Vueltas"=0, "Velocidad"=0, "Reserva1"=0, "Reserva2"=0}, "M_antebrazo"={"Pasos"=0, "Vueltas"=0, "Velocidad"=0, "Reserva1"=0, "Reserva2"=0}, "M_muneca"={"Pasos"=0, "Vueltas"=0, "Velocidad"=0, "Reserva1"=0, "Reserva2"=0}, "M_gripper"={"Pasos"=0, "Vueltas"=0, "Velocidad"=0, "Reserva1"=0, "Reserva2"=0}}, "Errores"={"Contador_correcto"=0, "Contador_errores"=0, "Edo_conex"=0}, "new_data?"=FALSE} ("Enc_values") T2 {"buffer"="", "Datos6_Motores"={"M_cadera"={"Pasos"=0, "Vueltas"=0, "Velocidad"=0, "Reserva1"=0, "Reserva2"=0}, "M_hombro"={"Pasos"=0, "Vueltas"=0, "Velocidad"=0, "Reserva1"=0, "Reserva2"=0}, "M_codo"={"Pasos"=0, "Vueltas"=0, "Velocidad"=0, "Reserva1"=0, "Reserva2"=0}, "M_antebrazo"={"Pasos"=0, "Vueltas"=0, "Velocidad"=0, "Reserva1"=0, "Reserva2"=0}, "M_muneca"={"Pasos"=0, "Vueltas"=0, "Velocidad"=0, "Reserva1"=0, "Reserva2"=0}, "M_gripper"={"Pasos"=0, "Vueltas"=0, "Velocidad"=0, "Reserva1"=0, "Reserva2"=0}}, "Errores"={"Contador_correcto"=0, "Contador_errores"=0, "Edo_conex"=0}, "new_data?"=FALSE} ("Enc_values") w379] -> w354
      tunnel: [w366 w370 w376] -> w348
      tunnel: w351 -> [w367 w371 w378]
      tunnel: [w367 w371 w378] -> w350
      tunnel: w349 -> [_ _ w377]
      tunnel: [TRUE FALSE w377] -> w347
      frame "Start" {
      }
      frame "Stop" {
      }
      frame "Idle", Default {
        # "Actualiza la UI constantemente"
        n106 = call "FGV_DatosMotores.vi"("error in (no error)"=w375, "Estado"=Ctrl_Fgv_DatosMotores."Get") -> ("error out"=w376:errorcluster, "Val_motor_out"=w379:T2)  [unwired: 8 in]
      }
    }
    n107 = call "actualizarIndicadores.vi"("error in (no error) 2"=w348, "indicator_cluster_in"=w352, "MotoresQueue_in"=w354) -> ("error out"=w346:errorcluster, "indicator_cluster_out"=w353:T10, "Errores.Edo_conex"=→"Serial errors":u32)  [unwired: 4 in, 2 out]
    n108 = call "FGV_Error.vi"("error_in_loop"=w346, "Estado"=enum16{"Set", "Get"}."Set") -> ("error out"=w343:errorcluster)  [unwired: 9 in]
    n109 = call "FGV_Error.vi"("error_in_loop"=w343, "Estado"=enum16{"Set", "Get"}."Get") -> ("error out"=w342:errorcluster)  [unwired: 9 in]
    "Error_out" <- w342
  }
  n110 = while {
    shift-right: [w383] -> w20
    shift-left: w9 -> [w392]
    shift-right: [w389] -> _
    shift-left: w36 -> [w391]
    shift-right: [w390] -> _
    shift-left: refnum<file> refnum ("refnum out") -> [w393]
    shift-right: [w386] -> w19
    shift-left: w10 -> [w387]
    tunnel: [w385] -> w26
    stop <- w385 stop-if-true
    # "DATA LOGGER"
    n111 = Dequeue Element(queue=w387, timeout in ms (-1)=-1, error in (no error)=w392) -> (queue out=w386:refnum<queue>, element=w396:T8, timed out?=w397:bool, error out=w398:errorcluster)
    n112 = case shown="False" w397 {
      tunnel: w396 -> [w400 w401]
      tunnel: [w399 Ctrl_Estados."Idle" ("Enum")] -> w395
      tunnel: [w400 w401] -> w394
      frame False {
        # "Hay datos en la cola"
        n113 = Unbundle By Name(w400) -> ("Estado"=w399:T6)
      }
      frame True {
        # "Timeout"
      }
    }
    n114 = case shown="\"Start\"" w395 {
      tunnel: w398 -> [w405 w409 w420 w465 w509]
      tunnel: [w405 w410 w418 w461 w501] -> w382
      tunnel: [FALSE TRUE FALSE FALSE FALSE] -> w385
      tunnel: w394 -> [_ _ w414 w460 _]
      tunnel: [w403 u32 0 ("millisecond timer value") w421 w464 w496] -> w389
      tunnel: [w404 refnum<file> refnum ("refnum out") w417 w462 w500] -> w390
      tunnel: w393 -> [w404 w408 w419 w466 _]
      tunnel: w391 -> [w403 _ w416 w458 _]
      frame "Idle", Default {
      }
      frame "Stop" {
        n115 = Close File(refnum=w408, error in=w409) -> (error out=w410:errorcluster)  [unwired: 1 out]
      }
      frame "Log_Data_All" {
        n116 = Unbundle By Name(w414) -> ("Enc_values.new_data?"=w413:bool)
        n117 = case shown="False" w413 {
          tunnel: w414 -> [_ w447]
          tunnel: [w422 w438] -> w421
          tunnel: w420 -> [w424 w437]
          tunnel: w419 -> [w423 w428]
          tunnel: [w424 w427] -> w418
          tunnel: [w423 w426] -> w417
          tunnel: w416 -> [w422 w425]
          frame False {
          }
          frame True {
            # "Hay nueva información"
            n118 = Unbundle By Name(w447) -> ("Enc_values.Datos6_Motores"=w446:T12)
            n119 = Unbundle By Name(w446) -> ("M_cadera"=w445:T3, "M_hombro"=w444:T3, "M_codo"=w443:T3, "M_antebrazo"=w442:T3, "M_muneca"=w441:T3, "M_gripper"=w440:T3)
            n120 = Build Array(w445, w444, w443, w442, w441, w440) -> (w439:T3[])
            n121 = for {
              tunnel: w439 -> [w457] mode=indexing
              tunnel: w437 -> [w451]
              tunnel: [w449] -> w436 mode=concatenating
              tunnel: [w448] -> w432
              n122 = Unbundle By Name(w457) -> ("Pasos"=w456:i32, "Vueltas"=w455:i16, "Velocidad"=w454:i16, "Reserva1"=w453:u8, "Reserva2"=w452:u8)
              n123 = Format Into String(format string="%d,%d,%d,%d,%d", error in=w451, w456, w455, w454, w453, w452) -> (resulting string=w449:string, error out=w448:errorcluster)  [unwired: 1 in]
            }
            n124 = Tick Count (ms)() -> (millisecond timer value=w438:u32)
            n125 = Subtract(x=w438, y=w425) -> (x-y=w433:u32)
            n126 = Format Into String(format string="%d,", error in=w432, w433) -> (resulting string=w434:string, error out=w430:errorcluster)  [unwired: 1 in]
            n127 = Concatenate Strings(w434, w436, "\\n" ("string")) -> (w429:string)
            n128 = Write to Text File(file (use dialog)=w428, text=w429, error in=w430) -> (refnum out=w426:refnum<file>, error out=w427:errorcluster)  [unwired: 1 in, 1 out]
          }
        }
      }
      frame "LogData" {
        n129 = Unbundle By Name(w460) -> ("Enc_values.new_data?"=w459:bool)
        n130 = case shown="False" w459 {
          tunnel: w466 -> [w468 w484]
          tunnel: w460 -> [_ w483]
          tunnel: w465 -> [w469 w482]
          tunnel: [w467 w481] -> w464
          tunnel: [w468 w480] -> w462
          tunnel: [w469 w479] -> w461
          tunnel: w458 -> [w467 w470]
          frame False {
            # "No registramos datos repetidos"
          }
          frame True {
            # "Hay nuevos datos"
            n131 = Unbundle By Name(w483) -> ("Enc_values.Datos6_Motores"=w492:T12)
            n132 = Unbundle By Name(w492) -> ("M_cadera"=w472:T3)
            n133 = Unbundle By Name(w472) -> ("Pasos"=w477:i32, "Vueltas"=w476:i16, "Velocidad"=w475:i16, "Reserva1"=w474:u8, "Reserva2"=w473:u8)
            n134 = Tick Count (ms)() -> (millisecond timer value=w481:u32)
            n135 = Format Into String(format string="%d,%d,%d,%d,%d", error in=w482, w477, w476, w475, w474, w473) -> (resulting string=w491:string, error out=w488:errorcluster)  [unwired: 1 in]
            n136 = Subtract(x=w481, y=w470) -> (x-y=w489:u32)
            n137 = Format Into String(format string="%d,", error in=w488, w489) -> (resulting string=w490:string, error out=w486:errorcluster)  [unwired: 1 in]
            n138 = Concatenate Strings(w490, w491, "\r\n") -> (w485:string)
            n139 = Write to Text File(file (use dialog)=w484, text=w485, error in=w486) -> (refnum out=w480:refnum<file>, error out=w479:errorcluster)  [unwired: 1 in, 1 out]
          }
        }
      }
      frame "Start" {
        n140 = Get Date/Time String() -> (time string=w512:string)  [unwired: 3 in, 1 out]
        n141 = Current VI's Path() -> (path=w515:path)
        n142 = Search and Replace String(input string=w512, search string=":", replace string="_" ("replace string (\"\")"), error in=w509) -> (result string=w495:string, error out=w505:errorcluster)  [unwired: 4 in, 2 out]
        n143 = Strip Path(path=w515) -> (stripped path=w514:path)  [unwired: 1 out]
        n144 = String Subset(string=w495, length (rest)=5 ("length (rest)")) -> (substring=w493:string)  [unwired: 1 in]
        n145 = Build Path(base path=w514, name or relative path=path "Excel") -> (appended path=w513:path)
        n146 = Concatenate Strings("test_" ("string"), w493, ".csv" ("string")) -> (w506:string)
        n147 = Build Path(base path=w513, name or relative path=w506) -> (appended path=w504:path)
        n148 = Concatenate Strings("Tiempo,C_Pas,C_Vue,C_Vel,C_R1,C_R2,H_Pas,H_Vue,H_Vel,H_R1,H_R2,Co_Pas,Co_Vue,Co_Vel,Co_R1,Co_R2,A_Pas,A_Vue,A_Vel,A_R1,A_R2,M_Pas,M_Vue,M_Vel,M_R1,M_R2,G_Pas,G_Vue,G_Vel,G_R1,G_R2" ("text"), "\r\n") -> (w497:string)
        n149 = Open/Create/Replace File(file path (use dialog)=w504, error in=w505, operation (0:open)=T11."open or create", access (0:read/write)=enum16{"read/write", "read-only", "write-only"}."read/write") -> (refnum out=w503:refnum<file>, error out=w502:errorcluster)  [unwired: 2 in, 1 out]
        n150 = Write to Text File(file (use dialog)=w503, text=w497, error in=w502) -> (refnum out=w500:refnum<file>, error out=w501:errorcluster)  [unwired: 1 in, 1 out]
        n151 = Tick Count (ms)() -> (millisecond timer value=w496:u32)
      }
    }
    n152 = call "FGV_Error.vi"("error_in_loop"=w382, "Estado"=enum16{"Set", "Get"}."Set") -> ("error out"=w383:errorcluster)  [unwired: 9 in]
  }
  n153 = Release Queue(queue=w18, error in (no error)=w17) -> ()  [unwired: 1 in, 3 out]
  n154 = Release Queue(queue=w19, error in (no error)=w20) -> ()  [unwired: 1 in, 3 out]
  n155 = Compound Arithmetic op=AND(w25, w27, w26, w24) -> (w28:bool)
  n156 = control-ref of="Start_ind"() -> (w34:refnum<vi>)
  n157 = property class="Bool"(reference=w34, "Value"=w28) -> ()  [unwired: 1 in, 2 out]
